vi "niFpgaDEN_MinimumSizeInfo.vi"() -> ()   [LabVIEW 2017]
panel:
  out "kDENMaxNDispChar":i32=100
  out "kDENFooterHeight":i32=10
  out "kDENMinHeight":i32=58
  out "kDENMinWidth":i32=96
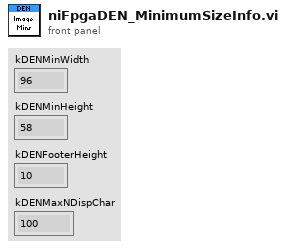
[diagram p1: front panel]
diagram:
